vi "Encoder Simulation.vi"() -> ()   [LabVIEW 2018]
uses:
  <vilib>/Simulation/Scripting/Companion Diagram/SimConfigNode/SimParams.ctl
  <vilib>/Simulation/Scripting/Companion Diagram/SimConfigNode/_simSolvers.ctl
  <vilib>/Simulation/Implementation/Shared/SIMSCR Execution Mode.ctl
  <vilib>/Simulation/Param Hierarchy/Typedefs/SIMPH Param Control Actions.ctl
  <vilib>/Simulation/Implementation/Shared/NILVSim_ParamChanged.vi
  <vilib>/Simulation/Implementation/Shared/NILVSIM_BeginStep.vi
  <vilib>/Simulation/SignalArithmetic/Implementation/NILVSim Gain.llb/SIM Gain (scalar).vi
  <vilib>/Simulation/DataSources/Implementation/NILVSim Pulse Generator.llb/SIM Pulse Generator (scalar).vi
  <vilib>/Simulation/Utility/Implementation/SIM Halt.vi
  <vilib>/Simulation/Implementation/Shared/NILVSim_Manager.vi
  <vilib>/Utility/error.llb/Clear Errors.vi
  <vilib>/Simulation/Implementation/Shared/NILVSim_FinalizeModel.vi
  <vilib>/Simulation/Implementation/Shared/SIM Unbundle Sim Info.vi
  <vilib>/Simulation/Implementation/Shared/NILVSim_Initialize.vi
  Bidirectional Quadrature Decoder .vi
  Unidirectional Quadrature Decoder.vi
  <vilib>/Simulation/Utility/Implementation/NILVSim Get Time and IsAcceptedStep.vi
  Bidirectional Quadrature Decoder with reset.vi
  <vilib>/Simulation/Implementation/Shared/SIMSH Read Queue.vi
  <vilib>/Simulation/Implementation/Shared/NILVSim_GetModelError.vi
  <vilib>/Simulation/Implementation/Shared/SIM Bundle Sim Info.vi
  <vilib>/Simulation/Scripting/Companion Diagram/SimConfigNode/SimDog.xnode
  <vilib>/Simulation/Implementation/XNodeFramework/SimXNode/SimX.xnode
  <vilib>/Simulation/Implementation/Shared/NI_SIM_Implementation.lvlib
panel:
  in  "Pulses Per Revolution (PPR)":dbl=512.0
  in  "Direction":enum16{"B leads A (CW)", "A leads B (CCW)"}(ring)=enum."A leads B (CCW)"
  out "# of counts":i32
  in  "Stop Button":bool
  in  "Reset":bool
  in  "Step Size (s)":dbl=0.1
  in  "Period (s)":dbl=1.0
  # "Mechatronic Systems Board"
  # "Mechatronic Systems Board"
  # "Encoder Simulation"
  # "Blob Detection"
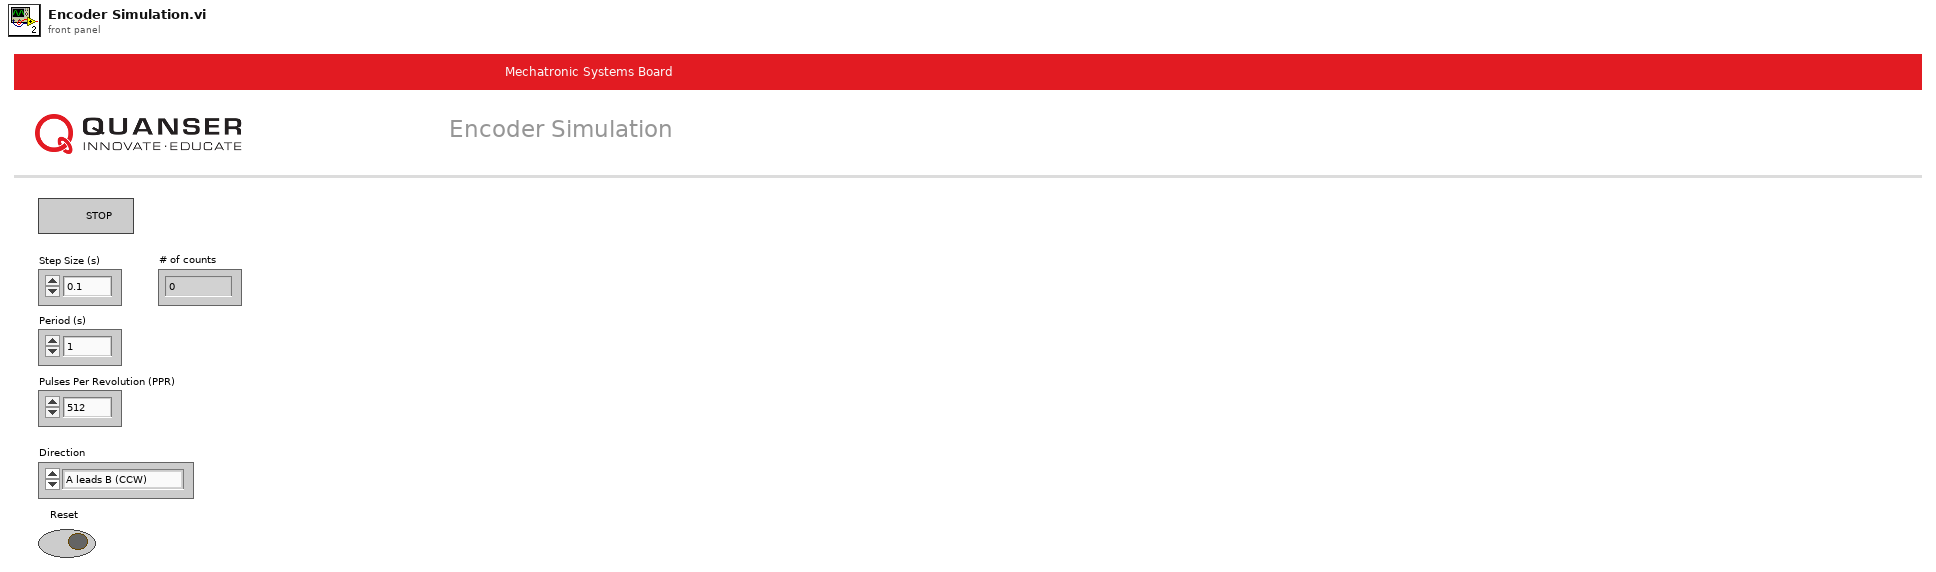
[diagram p1: front panel]
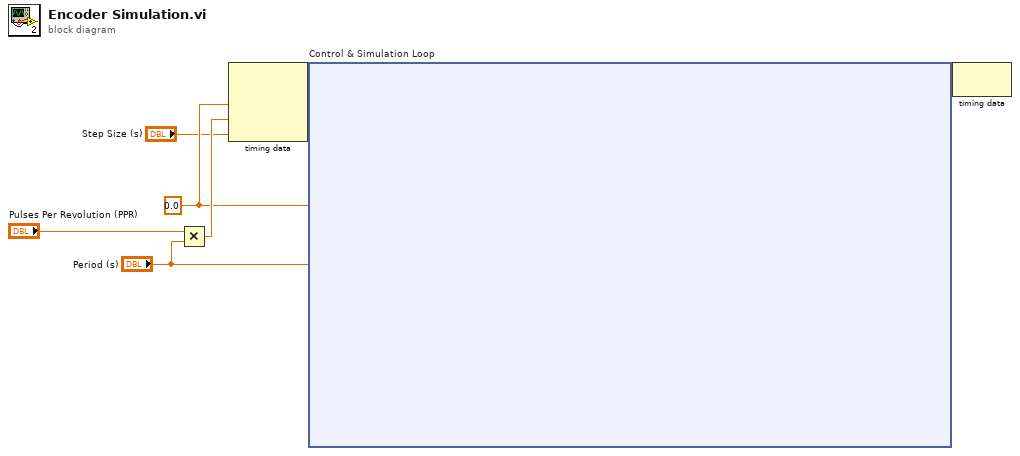
[diagram p0: block diagram]
diagram:
  w4 = 0.0 ("period 2")
  n1 = Multiply(x="Pulses Per Revolution (PPR)", y="Period (s)") -> (x*y=w5:dbl)
  n2 = node-c288(w4, w5, "Step Size (s)") -> (w7:variant)  [unwired: 1 in]
  n3 = node-c254 "Control & Simulation Loop"(w7, "Period (s)", w4) -> (w6:variant)
  n4 = node-c288(w6) -> ()  [unwired: 1 out]
